vi "tm_setarea.vi"(8 "error in (no error)":errorcluster, 10 "Sub Region":T1, 11 "Handle in":u32) -> (0 "error out":errorcluster, 3 "Handle out":u32)   [LabVIEW 2011]
uses:
  tmcamcon.dll
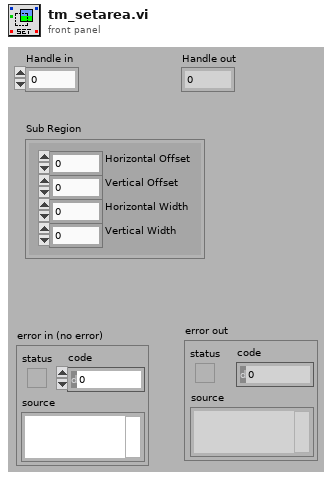
[diagram p1: front panel]
types:
  T1 = cluster{"Horizontal Offset":i32, "Vertical Offset":i32, "Horizontal Width":i32, "Vertical Width":i32}
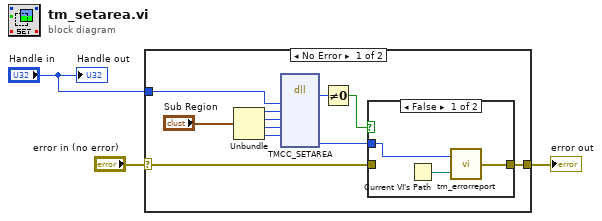
[diagram p0: block diagram]
diagram:
  n1 = case shown="No Error" "error in (no error)" {
    selector: "error in (no error)" -> [w7 w19]
    tunnel: [w4 w19] -> w2
    tunnel: "Handle in" -> [w8 _]
    frame No Error {
      n2 = Unbundle("Sub Region") -> ("Horizontal Offset"=w9:i32, "Vertical Offset"=w10:i32, "Horizontal Width"=w11:i32, "Vertical Width"=w12:i32)
      n3 = dll-call lib="tmcamcon.dll" fn="TMCC_SETAREA"("HDCAM"=w8, "sho"=w9, "svo"=w10, "shw"=w11, "svw"=w12) -> ("return type"=w14:u32, "Erval"=w6:i32)  [unwired: 9 in, 2 out]
      n4 = Not Equal To 0?(x=w14) -> (x != 0?=w5:bool)
      n5 = case shown="False" w5 {
        tunnel: w7 -> [_ w18]
        tunnel: [w16 w18] -> w4
        tunnel: w6 -> [w15 _]
        frame False {
          n6 = Current VI's Path() -> (path=w17:path)
          n7 = call <userlib>:"tm_errorreport.vi"("Source"=w17, "Error"=w15) -> ("error out"=w16:errorcluster)
        }
        frame True {
        }
      }
    }
    frame Error {
    }
  }
  "error out" <- w2
  "Handle out" <- "Handle in"
